vi "RM.removeNodeReservation.vi"(7 "Resource Type":T1, 8 "error in":errorcluster, 10 "name in bitfile":string, 11 "Item Ref in":T2 format="%.0x") -> (0 "error out":errorcluster, 2 "found":bool, 3 "Item Ref out":T2 format="%.0x")   [LabVIEW 2016, in "FPGA Resource Manager.lvlib"]
uses:
  FPGA Resource Manager.lvlib
  <vilib>/NI Veristand/Custom Device API/Custom Device Item Ref.ctl
  RM.resourceType.ctl
  <vilib>/NI VeriStand/Custom Device API/Custom Device API.lvlib
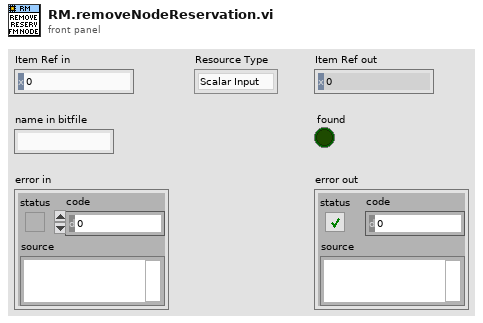
[diagram p1: front panel]
types:
  T1 = typedef "FPGA Resource Manager.lvlib/RM.resourceType.ctl" = enum16{"Scalar Input", "Scalar Output", "Waveform Input", "Waveform Output"}
  T2 = typedef "Custom Device API.lvlib/Custom Device Item Ref.ctl" = u64
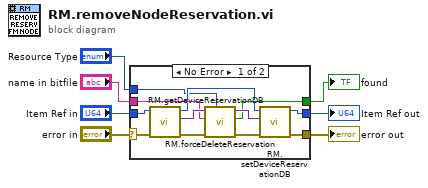
[diagram p0: block diagram]
diagram:
  n1 = case shown="No Error" "error in" {
    selector: "error in" -> [w15 w20]
    tunnel: "Item Ref in" -> [w16 w21]
    tunnel: [w14 w21] -> w5
    tunnel: [w13 w20] -> w4
    tunnel: [w12 _] -> w3
    tunnel: "name in bitfile" -> [w11 _]
    tunnel: "Resource Type" -> [w8 _]
    frame No Error {
      n2 = call "RM.getDeviceReservationDB.vi"("error in"=w15, "Item Ref in"=w16) -> ("error out"=w10:errorcluster, "reservation DB out"=w18:variant, "Item Ref out"=w9:T2)  [unwired: 6 in, 1 out]
      n3 = call "RM.forceDeleteReservation.vi"("Resource Type"=w8, "error in"=w10, "name in bitfile"=w11, "reservation DB in"=w18) -> ("error out"=w19:errorcluster, "found?"=w12:bool, "reservation DB out"=w17:variant)  [unwired: 5 in]
      n4 = call "RM.setDeviceReservationDB.vi"("error in"=w19, "reservation DB in"=w17, "Item Ref in"=w9) -> ("error out"=w13:errorcluster, "Item Ref out"=w14:T2)  [unwired: 6 in, 1 out]
    }
    frame Error {
    }
  }
  "Item Ref out" <- w5
  "error out" <- w4
  "found" <- w3
